vi "Compile and Export Settings.vi"(8 "error in (no error)":errorcluster, 11 "Device Item Ref in":T1 format="%.0x") -> (0 "error out":errorcluster)   [LabVIEW 2015, in "Protection and Rolling Counter Addon System Explorer.lvlib"]
uses:
  Protection and Rolling Counter Addon System Explorer.lvlib
  <vilib>/NI Veristand/Custom Device API/Custom Device Item Ref.ctl
  Shared/Types/Exported.OnCompile.ctl
  Shared/Types/XNET Settings.ctl
  Shared/Types/Exported Frame Settings.ctl
  Shared/Types/Exported Frame Type.ctl
  Shared/Types/Exported Protection Settings.ctl
  Shared/Types/Protection Type.ctl
  Shared/Types/InputChannelConfiguration.ctl
  Shared/Types/Exported Counter Settings.ctl
  Shared/Types/Event Trigger Type.ctl
  <vilib>/NI Veristand/Custom Device Tools/Custom Device Utility Library/Search Direction.ctl
  Shared/SubVIs/GUID Lookup.vi
  <vilib>/NI Veristand/Custom Device Tools/Custom Device Utility Library/NI VeriStand - Search for Item by GUID.vi
  <vilib>/NI Veristand/Custom Device Tools/Custom Device Utility Library/NI VeriStand - Search for All Items by GUID.vi
  <vilib>/NI Veristand/Custom Device API/Set Item Property (Variant).vi
  <vilib>/NI VeriStand/Custom Device Tools/Custom Device Utility Library/Custom Device Utility Library.lvlib
  Shared/Protection and Rolling Counter Addon Shared.lvlib
  <vilib>/NI VeriStand/Custom Device API/Custom Device API.lvlib
  <resource>/objmgr/xnet.rc
  <vilib>/NI/NIVS Inline Async API/_Data Access System Explorer/Data Access System Explorer.lvlib
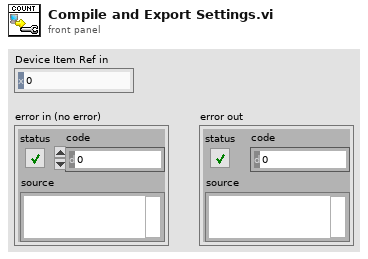
[diagram p1: front panel]
types:
  T1 = typedef "Custom Device API.lvlib/Custom Device Item Ref.ctl" = u64
  T2 = typedef "Custom Device Utility Library.lvlib/Search Direction.ctl" = enum16{"Down", "Up"}
  T3 = typedef "Protection and Rolling Counter Addon Shared.lvlib/Exported Frame Type.ctl" = enum16{"Periodic", "Event", "Periodic/Event"}
  T4 = typedef "Protection and Rolling Counter Addon Shared.lvlib/Exported Frame Settings.ctl" = cluster{"Type":T3, "Frame ID":u32, "Payload Length":u32, "Signal XNET Paths":string[], "Frame.PrevData":dbl[], "VS Offset":i32, "VS Length":i32, "Generation Period":u32, "Has Protection?":bool, "Protection Configurations":T5[], "Has Counter":bool, "Counter Configurations":T8[], "Has Disable?":bool, "Disable VS Index":i32, "Transmit Trigger":T9, "Trigger VS Index":i32}
  T5 = typedef "Protection and Rolling Counter Addon Shared.lvlib/Exported Protection Settings.ctl" = cluster{"Protection Frame Index":i32, "Protection Type":T6, "Data Indeces":i32[], "Initialized Data Array":dbl[], "Protection Signal XNET Paths":string[], "CRC Channels":T7[], "Protection VS Update Index":i32}
  T6 = typedef "Protection and Rolling Counter Addon Shared.lvlib/Protection Type.ctl" = enum16{"Arb ID + Bytes Checksum with Inversion", "Arb ID + Bytes CRC with Inversion", "Reversed Raw Signal Checksum with Inversion"}
  T7 = typedef "Protection and Rolling Counter Addon Shared.lvlib/InputChannelConfiguration.ctl" = cluster{"Start Bit":i32, "Name":string, "Number of bits":i32, "Scale":dbl, "Offset":dbl, "Data Type":u32}
  T8 = typedef "Protection and Rolling Counter Addon Shared.lvlib/Exported Counter Settings.ctl" = cluster{"Counter Frame Index":i32, "Max Count":dbl, "Counter VS Index":i32}
  T9 = typedef "Protection and Rolling Counter Addon Shared.lvlib/Event Trigger Type.ctl" = enum16{"Channel value change", "Trigger channel (not zero)", "Channel value change or trigger channel (not zero)", "Trigger channel (any value change)", "Channel value change or trigger channel (any value change)"}
  T10 = cluster{"Name":string, "Type":enum16{"Output/Write", "Input/Read", "Input/ReadWrite"}, "VS Refs":T1[]}
  T11 = typedef "Protection and Rolling Counter Addon Shared.lvlib/Exported.OnCompile.ctl" = cluster{"XNET Settings":T12, "Frames":T4[]}
  T12 = typedef "Protection and Rolling Counter Addon Shared.lvlib/XNET Settings.ctl" = cluster{"Database":refnum<k21>, "Cluster":refnum<k21>, "Port":string, "Baud rate [Bd]":u64, "Termination":u32, "CAN I/O Mode":u32, "FD Baud rate [Bd]":u64, "Priority":i32, "Use Legacy":bool}
  T13 = typedef "Custom Device API.lvlib/Custom Device Item Info.ctl" = cluster{"Name":string, "Is Channel":bool, "GUID":string, "Is Waveform":bool}
  T14 = typedef "Protection and Rolling Counter Addon System Explorer.lvlib/Frame Settings.ctl" = cluster{"ID":u32, "Disable Transmission":bool, "Disable Transmission Ref":T1, "Transmit Trigger":T9, "Transmit Trigger Ref":T1}
  T15 = typedef "Protection and Rolling Counter Addon System Explorer.lvlib/Protection Signal Settings.ctl" = cluster{"Input Channels":T16[], "Protection Type":T6}
  T16 = typedef "Protection and Rolling Counter Addon System Explorer.lvlib/Protection Signal Linked Channels.ctl" = cluster{"Node Ref":T1}
  T17 = cluster{"Name":string, "Type":enum16{"Output/Write", "Input/Read", "Input/ReadWrite"}, "VS Refs":T1[]}[]
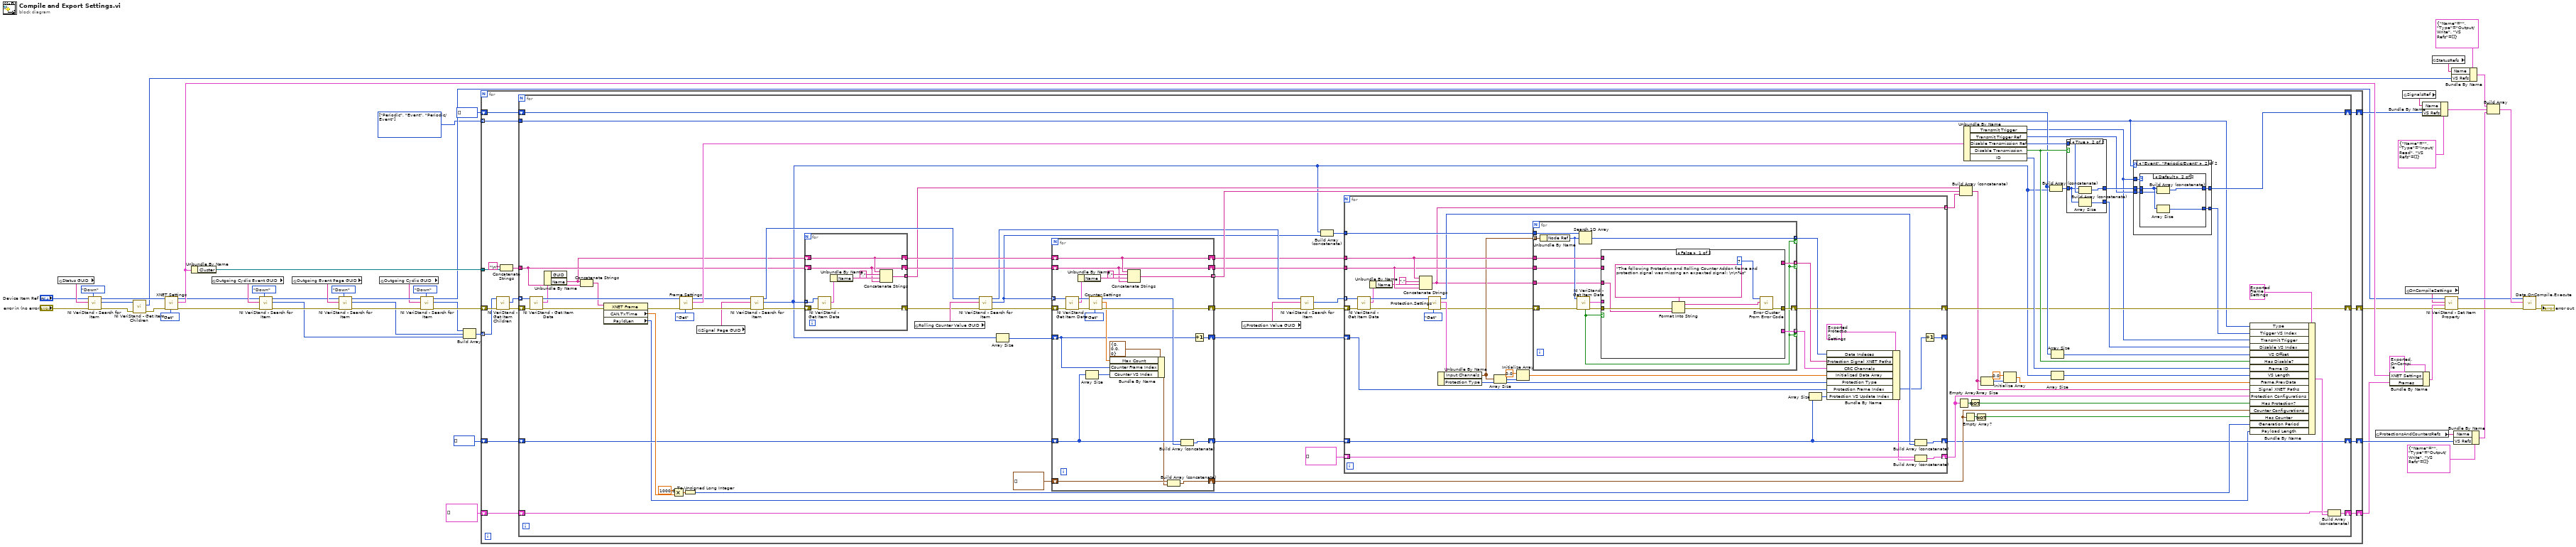
[diagram p0: block diagram]
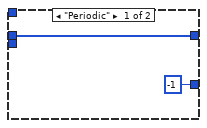
[diagram p2: hidden frame]
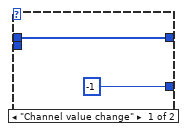
[diagram p3: hidden frame]
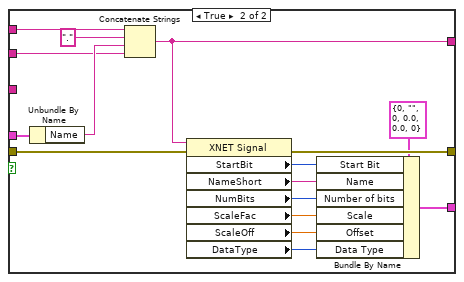
[diagram p4: hidden frame]
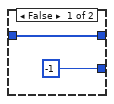
[diagram p5: hidden frame]
diagram:
  w11 = T3[] [enum."Periodic", enum."Event", enum."Periodic/Event"] items=["Periodic", "Event", "Periodic/Event"]
  n1 = global read "GUID Lookup.vi" "Status GUID"() -> (w29:string)
  n2 = call-poly <vilib>:"NI VeriStand - Search for Item.vi"("Direction (Down)"=Search_Direction."Down", "error in"="error in (no error)", "Item GUID"=w29, "Section Ref in"="Device Item Ref in") -> ("error out"=w24:errorcluster, "Item Ref"=w25:T1, "Section Ref out"=w26:T1)  [unwired: 4 in, 1 out]
  n3 = call <vilib>:"NI VeriStand - Get Item Children.vi"("error in (no error)"=w24, "Item Ref in"=w25) -> ("error out"=w23:errorcluster, "Child Refs"=w22:T1[])  [unwired: 6 in, 2 out]
  n4 = call "XNET.Settings.vi"("Action"=enum8{"Get", "Set"}."Get", "error in (no error)"=w23, "Parent Ref in"=w26) -> ("error out"=w5:errorcluster, "XNET Settings"=w49:T12, "Item Ref out"=w4:T1)  [unwired: 6 in]
  n5 = Unbundle By Name(w49) -> ("Cluster"=w51:refnum<k21>)
  n6 = global read "GUID Lookup.vi" "Outgoing Cyclic Event GUID"() -> (w7:string)
  n7 = call-poly <vilib>:"NI VeriStand - Search for Item.vi"("Direction (Down)"=Search_Direction."Down", "error in"=w5, "Item GUID"=w7, "Section Ref in"=w4) -> ("error out"=w2:errorcluster, "Item Ref"=w1:T1, "Section Ref out"=w3:T1)  [unwired: 4 in, 1 out]
  n8 = global read "GUID Lookup.vi" "Outgoing Event Page GUID"() -> (w13:string)
  n9 = call-poly <vilib>:"NI VeriStand - Search for Item.vi"("Direction (Down)"=Search_Direction."Down", "error in"=w2, "Item GUID"=w13, "Section Ref in"=w3) -> ("error out"=w19:errorcluster, "Item Ref"=w17:T1, "Section Ref out"=w20:T1)  [unwired: 4 in, 1 out]
  n10 = global read "GUID Lookup.vi" "Outgoing Cyclic GUID"() -> (w12:string)
  n11 = call-poly <vilib>:"NI VeriStand - Search for Item.vi"("Direction (Down)"=Search_Direction."Down", "error in"=w19, "Item GUID"=w12, "Section Ref in"=w20) -> ("error out"=w53:errorcluster, "Item Ref"=w18:T1, "Section Ref out"=w41:T1)  [unwired: 4 in, 1 out]
  n12 = Build Array(w18, w17, w1) -> (w16:T1[])
  n13 = for {
    tunnel: w51 -> [w66]
    shift-right: [w61] -> w40
    shift-left: w53 -> [w69]
    tunnel: w16 -> [w60] mode=indexing
    shift-right: [w59] -> w15
    shift-left: T4[] [] -> [w58]
    tunnel: w11 -> [w57] mode=indexing
    shift-right: [w63] -> w46
    shift-left: T1[] [] -> [w56]
    shift-right: [w62] -> w42
    shift-left: T1[] [] -> [w55]
    n14 = call <vilib>:"NI VeriStand - Get Item Children.vi"("error in (no error)"=w69, "Item Ref in"=w60) -> ("error out"=w67:errorcluster, "Child Refs"=w68:T1[])  [unwired: 6 in, 2 out]
    n15 = Concatenate Strings("\n", w66) -> (w64:string)
    n16 = for {
      tunnel: w68 -> [w123] mode=indexing
      shift-right: [w87] -> w61
      shift-left: w67 -> [w124]
      shift-right: [w135] -> w63
      shift-left: w56 -> [w133]
      tunnel: w64 -> [w104]
      shift-right: [w81] -> w62
      shift-left: w55 -> [w112]
      shift-right: [w72] -> w59
      shift-left: w58 -> [w71]
      tunnel: w57 -> [w70]
      n17 = call <vilib>:"NI VeriStand - Get Item Data.vi"("error in (no error)"=w124, "Item Ref in"=w123) -> ("error out"=w119:errorcluster, "Item Info"=w121:T13, "Item Ref out"=w122:T1)  [unwired: 6 in, 1 out]
      n18 = Unbundle By Name(w121) -> ("Name"=w103:string)  [unwired: 1 out]
      n19 = Concatenate Strings(w103, w104) -> (w120:string)
      n20 = property class="XNET Frame"(reference=w120, error in=w119) -> (error out=w118:errorcluster, "CAN.TxTime"=w116:dbl, "PayldLen"=w77:u32)  [unwired: 1 out]
      n21 = Multiply(x=1000.0 ("y"), y=w116) -> (x*y=w117:dbl)
      n22 = call "Frame.Settings.vi"("Action"=enum8{"Get", "Set"}."Get", "error in (no error)"=w118, "Item Ref in"=w122) -> ("error out"=w141:errorcluster, "Frame.Settings"=w142:T14, "Item Ref out"=w139:T1)  [unwired: 6 in]
      n23 = To Unsigned Long Integer(number=w117) -> (unsigned 32bit integer=w114:u32)
      n24 = global read "GUID Lookup.vi" "Signal Page GUID"() -> (w111:string)
      n25 = call-poly <vilib>:"NI VeriStand - Search for Item.vi"("error in"=w141, "Item GUID"=w111, "Section Ref in"=w139) -> ("error out"=w106:errorcluster, "Item Refs"=w79:T1[], "Section Ref out"=w109:T1)  [unwired: 5 in, 1 out]
      n26 = for {
        tunnel: w79 -> [w236] mode=indexing
        shift-right: [w230] -> w105
        shift-left: w106 -> [w235]
        tunnel: [w232] -> w100 mode=indexing
        shift-right: [w229] -> w102
        shift-left: w103 -> [w229]
        shift-right: [w228] -> w101
        shift-left: w104 -> [w228]
        n27 = call <vilib>:"NI VeriStand - Get Item Data.vi"("error in (no error)"=w235, "Item Ref in"=w236) -> ("error out"=w230:errorcluster, "Item Info"=w231:T13)  [unwired: 6 in, 2 out]
        n28 = Unbundle By Name(w231) -> ("Name"=w233:string)
        n29 = Concatenate Strings(w229, "." ("string"), w233, w228) -> (w232:string)
      }
      n30 = global read "GUID Lookup.vi" "Rolling Counter Value GUID"() -> (w110:string)
      n31 = call-poly <vilib>:"NI VeriStand - Search for Item.vi"("error in"=w105, "Item GUID"=w110, "Section Ref in"=w109) -> ("error out"=w108:errorcluster, "Item Refs"=w78:T1[], "Section Ref out"=w96:T1)  [unwired: 5 in, 1 out]
      n32 = Array Size(array=w79) -> (size(s)=w107:i32)
      n33 = for {
        tunnel: w78 -> [w259] mode=indexing
        shift-right: [w253] -> w97
        shift-left: w108 -> [w258]
        shift-right: [w255] -> w125
        shift-left: T8[] [] -> [w254]
        tunnel: [w250] -> w99 mode=indexing
        shift-right: [w247] -> w82
        shift-left: w112 -> [w248]
        shift-right: [w240] -> w92
        shift-left: w107 -> [w241]
        shift-right: [w239] -> w90
        shift-left: w102 -> [w239]
        shift-right: [w238] -> w91
        shift-left: w101 -> [w238]
        n34 = call <vilib>:"NI VeriStand - Get Item Data.vi"("error in (no error)"=w258, "Item Ref in"=w259) -> ("error out"=w256:errorcluster, "Item Info"=w249:T13, "Item Ref out"=w257:T1)  [unwired: 6 in, 1 out]
        n35 = Unbundle By Name(w249) -> ("Name"=w251:string)
        n36 = Array Size(array=w248) -> (size(s)=w242:i32)
        n37 = call "Counter.Settings.vi"("Action"=enum8{"Get", "Set"}."Get", "error in"=w256, "Parent Ref"=w257) -> ("error out"=w253:errorcluster, "Max Count"=w246:dbl, "Parent Ref Out"=w243:T1)  [unwired: 6 in]
        n38 = Bundle By Name(cluster=T8 {"Counter Frame Index"=0, "Max Count"=0.0, "Counter VS Index"=0} ("Cluster"), "Max Count"=w246, "Counter Frame Index"=w241, "Counter VS Index"=w242) -> (w245:T8)
        n39 = Concatenate Strings(w239, "." ("string"), w251, w238) -> (w250:string)
        n40 = Build Array (concatenate)(w254, w245) -> (w255:T8[])
        n41 = Build Array (concatenate)(w248, w243) -> (w247:T1[])
        n42 = Increment(x=w241) -> (x+1=w240:i32)
      }
      n43 = global read "GUID Lookup.vi" "Protection Value GUID"() -> (w98:string)
      n44 = call-poly <vilib>:"NI VeriStand - Search for Item.vi"("error in"=w97, "Item GUID"=w98, "Section Ref in"=w96) -> ("error out"=w95:errorcluster, "Item Refs"=w94:T1[])  [unwired: 5 in, 2 out]
      n45 = Build Array (concatenate)(w79, w78) -> (w80:T1[])
      n46 = for {
        tunnel: w94 -> [w190] mode=indexing
        shift-right: [w183] -> w87
        shift-left: w95 -> [w189]
        shift-right: [w184] -> w88
        shift-left: T5[] [] -> [w186]
        tunnel: w80 -> [w185]
        tunnel: w90 -> [w181]
        tunnel: [w159] -> w89 mode=indexing
        shift-right: [w177] -> w81
        shift-left: w82 -> [w178]
        shift-right: [w161] -> _
        shift-left: w92 -> [w162]
        tunnel: w91 -> [w180]
        n47 = call <vilib>:"NI VeriStand - Get Item Data.vi"("error in (no error)"=w189, "Item Ref in"=w190) -> ("error out"=w187:errorcluster, "Item Info"=w179:T13, "Item Ref out"=w188:T1)  [unwired: 6 in, 1 out]
        n48 = Unbundle By Name(w179) -> ("Name"=w160:string)
        n49 = Concatenate Strings(w181, "." ("string"), w160, w180) -> (w159:string)
        n50 = call "Protection.Settings.vi"("Action"=enum8{"Get", "Set"}."Get", "error in"=w187, "Parent Ref"=w188) -> ("error out"=w167:errorcluster, "Selected Channels"=w176:T15, "Parent Ref Out"=w163:T1)  [unwired: 6 in]
        n51 = Unbundle By Name(w176) -> ("Input Channels"=w173:T16[], "Protection Type"=w175:T6)
        n52 = Array Size(array=w173) -> (size(s)=w172:i32)
        n53 = Initialize Array(0.0 ("element"), w172) -> (w170:dbl[])
        n54 = for {
          tunnel: w185 -> [w194]
          tunnel: w173 -> [w204] mode=indexing
          tunnel: [w203] -> w174 mode=indexing if=w192
          shift-right: [w197] -> w183
          shift-left: w167 -> [w202]
          tunnel: w181 -> [w200]
          tunnel: w180 -> [w199]
          tunnel: [w195] -> w166 mode=indexing if=w192
          tunnel: [w196] -> w168 mode=indexing if=w192
          tunnel: w159 -> [w191]
          n55 = Unbundle By Name(w204) -> ("Node Ref"=w193:T1)
          n56 = call <vilib>:"NI VeriStand - Get Item Data.vi"("error in (no error)"=w202, "Item Ref in"=w193) -> ("error out"=w198:errorcluster, "Item Info"=w201:T13, "Found"=w192:bool)  [unwired: 6 in, 1 out]
          n57 = Search 1D Array(1D array=w194, element=w193) -> (index of element=w203:i32)  [unwired: 1 in]
          n58 = case shown="False" w192 {
            tunnel: w201 -> [_ w227]
            tunnel: w200 -> [_ w224]
            tunnel: w199 -> [_ w223]
            tunnel: w198 -> [w209 w222]
            tunnel: [w211 w221] -> w197
            tunnel: [_ w213] -> w196
            tunnel: [_ w212] -> w195
            tunnel: w191 -> [w206 _]
            frame False {
              n59 = Format Into String(format string="The following Protection and Rolling Counter Addon frame and protection signal was missing an expexted signal: \n\n%s" ("error message (\"\")"), error in=w209, w206) -> (resulting string=w205:string, error out=w208:errorcluster)  [unwired: 1 in]
              n60 = call <vilib>:"Error Cluster From Error Code.vi"("error in (no error)"=w208, "error message (\"\")"=w205, "error code (0)"=7) -> ("error out"=w211:errorcluster)  [unwired: 6 in]
            }
            frame True {
              n61 = Unbundle By Name(w227) -> ("Name"=w225:string)
              n62 = Concatenate Strings(w224, "." ("string"), w225, w223) -> (w212:string)
              n63 = property class="XNET Signal"(reference=w212, error in=w222) -> (error out=w221:errorcluster, "StartBit"=w214:u32, "NameShort"=w215:string, "NumBits"=w216:u32, "ScaleFac"=w217:dbl, "ScaleOff"=w218:dbl, "DataType"=w219:u32)  [unwired: 1 out]
              n64 = Bundle By Name(cluster=T7 {"Start Bit"=0, "Name"="", "Number of bits"=0, "Scale"=0.0, "Offset"=0.0, "Data Type"=0} ("MonitoredChannelSettings"), "Start Bit"=w214, "Name"=w215, "Number of bits"=w216, "Scale"=w217, "Offset"=w218, "Data Type"=w219) -> (w213:T7)
            }
          }
        }
        n65 = Array Size(array=w178) -> (size(s)=w164:i32)
        n66 = Bundle By Name(cluster=T5 {"Protection Frame Index"=0, "Protection Type"=enum."Arb ID + Bytes Checksum with Inversion", "Data Indeces"=[], "Initialized Data Array"=[], "Protection Signal XNET Paths"=[], "CRC Channels"=[], "Protection VS Update Index"=0} ("Cluster"), "Data Indeces"=w174, "Protection Signal XNET Paths"=w166, "CRC Channels"=w168, "Initialized Data Array"=w170, "Protection Type"=w175, "Protection Frame Index"=w162, "Protection VS Update Index"=w164) -> (w169:T5)
        n67 = Build Array (concatenate)(w178, w163) -> (w177:T1[])
        n68 = Build Array (concatenate)(w186, w169) -> (w184:T5[])
        n69 = Increment(x=w162) -> (x+1=w161:i32)
      }
      n70 = Empty Array?(array=w88) -> (empty?=w127:bool)
      n71 = Build Array (concatenate)(w100, w99, w89) -> (w86:string[])
      n72 = Unbundle By Name(w142) -> ("Transmit Trigger"=w75:T9, "Transmit Trigger Ref"=w76:T1, "Disable Transmission Ref"=w137:T1, "Disable Transmission"=w138:bool, "ID"=w140:u32)
      n73 = Empty Array?(array=w125) -> (empty?=w129:bool)
      n74 = Not(x=w127) -> (.not. x?=w126:bool)
      n75 = Not(x=w129) -> (.not. x?=w128:bool)
      n76 = Array Size(array=w86) -> (size(s)=w84:i32)
      n77 = Initialize Array(0.0 ("element"), w84) -> (w83:dbl[])
      n78 = Build Array (concatenate)(w133, w79) -> (w134:T1[])
      n79 = Array Size(array=w133) -> (size(s)=w132:i32)
      n80 = Array Size(array=w79) -> (size(s)=w113:i32)
      n81 = case shown="True" w138 {
        tunnel: w134 -> [w261 w263]
        tunnel: [w261 w265] -> w136
        tunnel: w137 -> [_ w264]
        tunnel: [-1 w262] -> w131
        frame False {
        }
        frame True {
          n82 = Build Array (concatenate)(w263, w264) -> (w265:T1[])
          n83 = Array Size(array=w263) -> (size(s)=w262:i32)
        }
      }
      n84 = case shown="\"Event\", \"Periodic/Event\"" w70 {
        tunnel: w136 -> [w146 w151]
        tunnel: [w146 w150] -> w135
        tunnel: w76 -> [_ w149]
        tunnel: w75 -> [_ w148]
        tunnel: [-1 w147] -> w74
        frame "Periodic" {
        }
        frame "Event", "Periodic/Event" {
          n85 = case shown="Default" w148 {
            tunnel: w151 -> [w153 w156]
            tunnel: [w153 w157] -> w150
            tunnel: [-1 w155] -> w147
            tunnel: w149 -> [_ w154]
            frame "Channel value change" {
            }
            frame Default {
              n86 = Array Size(array=w156) -> (size(s)=w155:i32)
              n87 = Build Array (concatenate)(w156, w154) -> (w157:T1[])
            }
          }
        }
      }
      n88 = Bundle By Name(cluster=T4 {"Type"=enum."Periodic", "Frame ID"=0, "Payload Length"=0, "Signal XNET Paths"=[], "Frame.PrevData"=[], "VS Offset"=0, "VS Length"=0, "Generation Period"=0, "Has Protection?"=FALSE, "Protection Configurations"=[], "Has Counter"=FALSE, "Counter Configurations"=[], "Has Disable?"=FALSE, "Disable VS Index"=0, "Transmit Trigger"=enum."Channel value change", "Trigger VS Index"=0} ("Frame Settings"), "Type"=w70, "Trigger VS Index"=w74, "Transmit Trigger"=w75, "Disable VS Index"=w131, "VS Offset"=w132, "Has Disable?"=w138, "Frame ID"=w140, "VS Length"=w113, "Frame.PrevData"=w83, "Signal XNET Paths"=w86, "Protection Configurations"=w88, "Has Protection?"=w126, "Counter Configurations"=w125, "Has Counter"=w128, "Generation Period"=w114, "Payload Length"=w77) -> (w73:T4)
      n89 = Build Array (concatenate)(w71, w73) -> (w72:T4[])
    }
  }
  n90 = global read "GUID Lookup.vi" "ProtectionsAndCountersRefs"() -> (w36:string)
  n91 = Bundle By Name(cluster=T11 {"XNET Settings"={"Database"="", "Cluster"="", "Port"="", "Baud rate [Bd]"=500000, "Termination"=1, "CAN I/O Mode"=0, "FD Baud rate [Bd]"=500000, "Priority"=100, "Use Legacy"=FALSE}, "Frames"=[]}, "XNET Settings"=w49, "Frames"=w15) -> (w48:T11)
  n92 = global read "GUID Lookup.vi" "SignalsRef"() -> (w37:string)
  n93 = global read "GUID Lookup.vi" "OnCompileSettings"() -> (w35:string)
  n94 = Bundle By Name(cluster=T10 {"Name"="", "Type"=enum."Input/Read", "VS Refs"=[]} ("Group"), "Name"=w37, "VS Refs"=w46) -> (w45:T10)
  n95 = global read "GUID Lookup.vi" "StatusRefs"() -> (w32:string)
  n96 = call-poly <vilib>:"NI VeriStand - Set Item Property.vi"("error in (no error)"=w40, "Value"=w48, "Property Name"=w35, "Item Ref in"=w41) -> ("error out"=w39:errorcluster, "Item Ref out"=w38:T1)  [unwired: 5 in, 1 out]
  n97 = Bundle By Name(cluster=T10 {"Name"="", "Type"=enum."Output/Write", "VS Refs"=[]} ("Group"), "Name"=w32, "VS Refs"=w22) -> (w31:T10)
  n98 = Bundle By Name(cluster=T10 {"Name"="", "Type"=enum."Output/Write", "VS Refs"=[]} ("Group"), "Name"=w36, "VS Refs"=w42) -> (w34:T10)
  n99 = Build Array(w31, w45, w34) -> (w44:T17)
  n100 = call <vilib>:"Data.OnCompile.Execute.vi"("error in"=w39, "VS Ref Groups"=w44, "Custom Device Ref"=w38) -> ("error out"=→"error out":errorcluster)  [unwired: 7 in, 1 out]
